vi "File_ExcludePaths.vi"(1 "Search paths":path[](array[path]), 3 "Exclude paths":path[](array[path]), 7 "Exceptions":string[](array[string])) -> (15 "Remaining paths":path[](array[path]), 17 "Excluded paths":path[](array[path]))   [LabVIEW 2010]
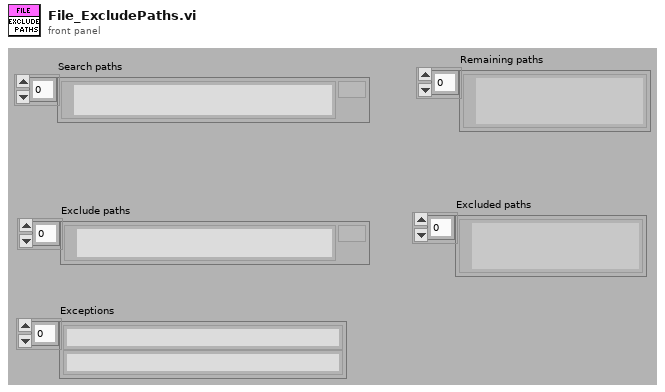
[diagram p1: front panel]
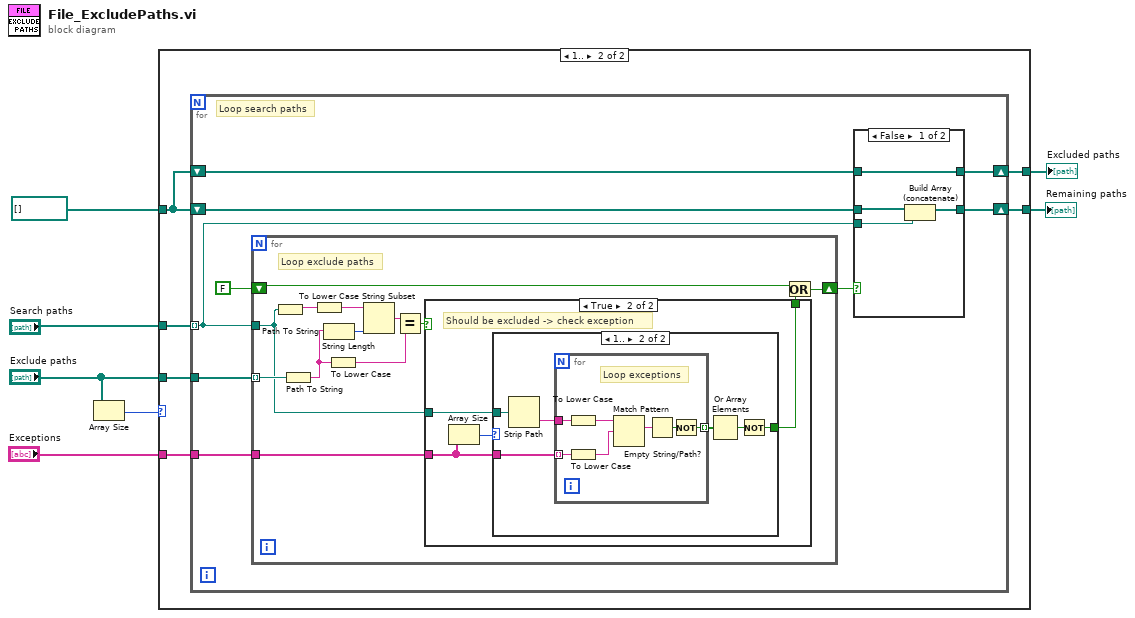
[diagram p0: block diagram]
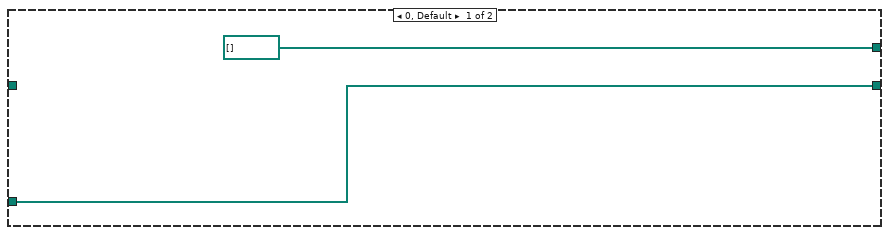
[diagram p2: hidden frame]
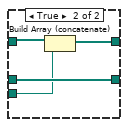
[diagram p3: hidden frame]
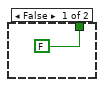
[diagram p4: hidden frame]
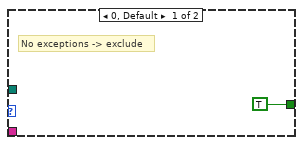
[diagram p5: hidden frame]
diagram:
  n1 = Array Size(array="Exclude paths") -> (size(s)=w3:i32)
  n2 = case shown="1.." w3 {
    tunnel: "Search paths" -> [w9 w15]
    tunnel: [w9 w14] -> w6
    tunnel: path[] [] ("Search paths") -> [_ w11]
    tunnel: "Exclude paths" -> [_ w13]
    tunnel: "Exceptions" -> [_ w12]
    tunnel: [path[] [] ("Search paths") w10] -> w1
    frame 0, Default {
    }
    frame 1.. {
      n3 = for {
        tunnel: w15 -> [w20] mode=indexing
        shift-right: [w21] -> w14
        shift-left: w11 -> [w22]
        tunnel: w13 -> [w24]
        tunnel: w12 -> [w18]
        shift-right: [w16] -> w10
        shift-left: w11 -> [w17]
        # "Loop search paths"
        n4 = for {
          tunnel: w20 -> [w37]
          tunnel: w24 -> [w41] mode=indexing
          shift-right: [w40] -> w19
          shift-left: FALSE -> [w39]
          tunnel: w18 -> [w38]
          # "Loop exclude paths"
          n5 = Path To String(path=w37) -> (string=w44:string)
          n6 = Path To String(path=w41) -> (string=w42:string)
          n7 = To Lower Case(string=w44) -> (all lower case string=w34:string)
          n8 = String Length(string=w42) -> (length=w45:i32)
          n9 = To Lower Case(string=w42) -> (all lower case string=w33:string)
          n10 = String Subset(string=w34, length (rest)=w45) -> (substring=w43:string)  [unwired: 1 out]
          n11 = Equal?(x=w43, y=w33) -> (x = y?=w36:bool)
          n12 = case shown="True" w36 {
            tunnel: w38 -> [_ w48]
            tunnel: w37 -> [_ w50]
            tunnel: [FALSE w49] -> w35
            frame False {
            }
            frame True {
              # "Should be excluded -> check exception"
              n13 = Array Size(array=w48) -> (size(s)=w47:i32)
              n14 = case shown="1.." w47 {
                tunnel: w48 -> [_ w57]
                tunnel: w50 -> [_ w56]
                tunnel: [TRUE w52] -> w49
                frame 0, Default {
                  # "No exceptions -> exclude"
                }
                frame 1.. {
                  n15 = Strip Path(path=w56) -> (name=w55:string)  [unwired: 1 out]
                  n16 = for {
                    tunnel: w57 -> [w63] mode=indexing
                    tunnel: w55 -> [w64]
                    tunnel: [w60] -> w54 mode=indexing
                    # "Loop exceptions"
                    n17 = To Lower Case(string=w64) -> (all lower case string=w59:string)
                    n18 = To Lower Case(string=w63) -> (all lower case string=w58:string)
                    n19 = Match Pattern(string=w59, regular expression=w58) -> (match substring=w62:string)  [unwired: 4 out]
                    n20 = Empty String/Path?(string/path=w62) -> (empty?=w61:bool)
                    n21 = Not(x=w61) -> (.not. x?=w60:bool)
                  }
                  n22 = Or Array Elements(Boolean array=w54) -> (logical OR=w53:bool)
                  n23 = Not(x=w53) -> (.not. x?=w52:bool)
                }
              }
            }
          }
          n24 = Or(x=w39, y=w35) -> (x .or. y?=w40:bool)
        }
        n25 = case shown="False" w19 {
          tunnel: w22 -> [w27 w32]
          tunnel: [w26 w32] -> w21
          tunnel: w20 -> [w28 w29]
          tunnel: w17 -> [w25 w31]
          tunnel: [w25 w30] -> w16
          frame False {
            n26 = Build Array (concatenate)(w27, w28) -> (w26:path[])
          }
          frame True {
            n27 = Build Array (concatenate)(w31, w29) -> (w30:path[])
          }
        }
      }
    }
  }
  "Remaining paths" <- w6
  "Excluded paths" <- w1
